vi "Get ObjFlags.vi"(8 "error in (no error)":errorcluster, 11 "OD Entry in":refnum<class "OD Entry.lvclass">) -> (0 "error out":errorcluster, 2 "ObjFlags":u32, 3 "OD Entry out":refnum<class "OD Entry.lvclass">)   [LabVIEW 2024, in "EDS.lvlib" / "OD Entry.lvclass"]
uses:
  OD Entry.lvclass
  OD Entry.lvclass/OD Entry.ctl
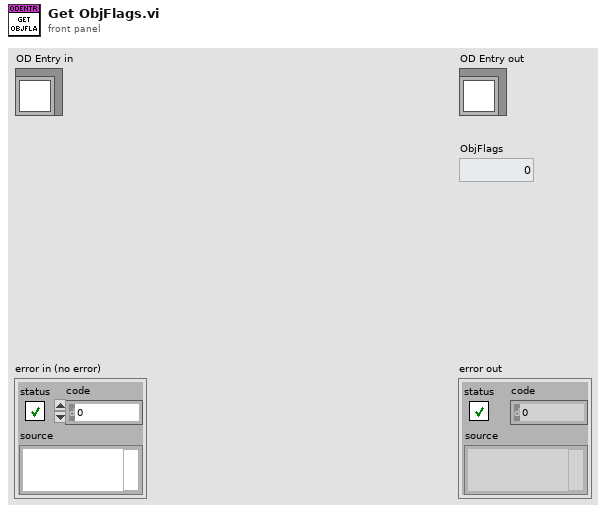
[diagram p1: front panel]
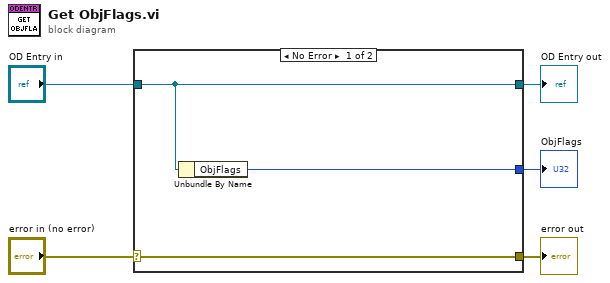
[diagram p0: block diagram]
diagram:
  n1 = case shown="No Error" "error in (no error)" {
    selector: "error in (no error)" -> [w8 w9]
    tunnel: [w8 w9] -> w4
    tunnel: [w7 w10] -> w2
    tunnel: "OD Entry in" -> [w7 w10]
    tunnel: [w6 _] -> w1
    frame No Error {
      n2 = Unbundle By Name(w7) -> ("ObjFlags"=w6:u32)
    }
    frame Error {
    }
  }
  "error out" <- w4
  "OD Entry out" <- w2
  "ObjFlags" <- w1
